vi "数组插入组合.vi"(10 "排序后的一维数组":string[](array[string]), 11 "输入数组":string[][](array[string])) -> (3 "输出结果":string[][](array[string]))   [LabVIEW 2016, in "数据传输系统.lvlib"]
uses:
  <userlib>/_OpenG.lib/array/array.llb/Search 1D Array (String)__ogtk.vi
  <userlib>/_OpenG.lib/array/array.llb/Delete Elements from 2D Array (String)__ogtk.vi
panel:
  out "数组列数":i32
  out "数组":string[][](array[string])
  out "禁用的索引 (列)":i32
  out "Indices of Elements":i32[](array[numeric])
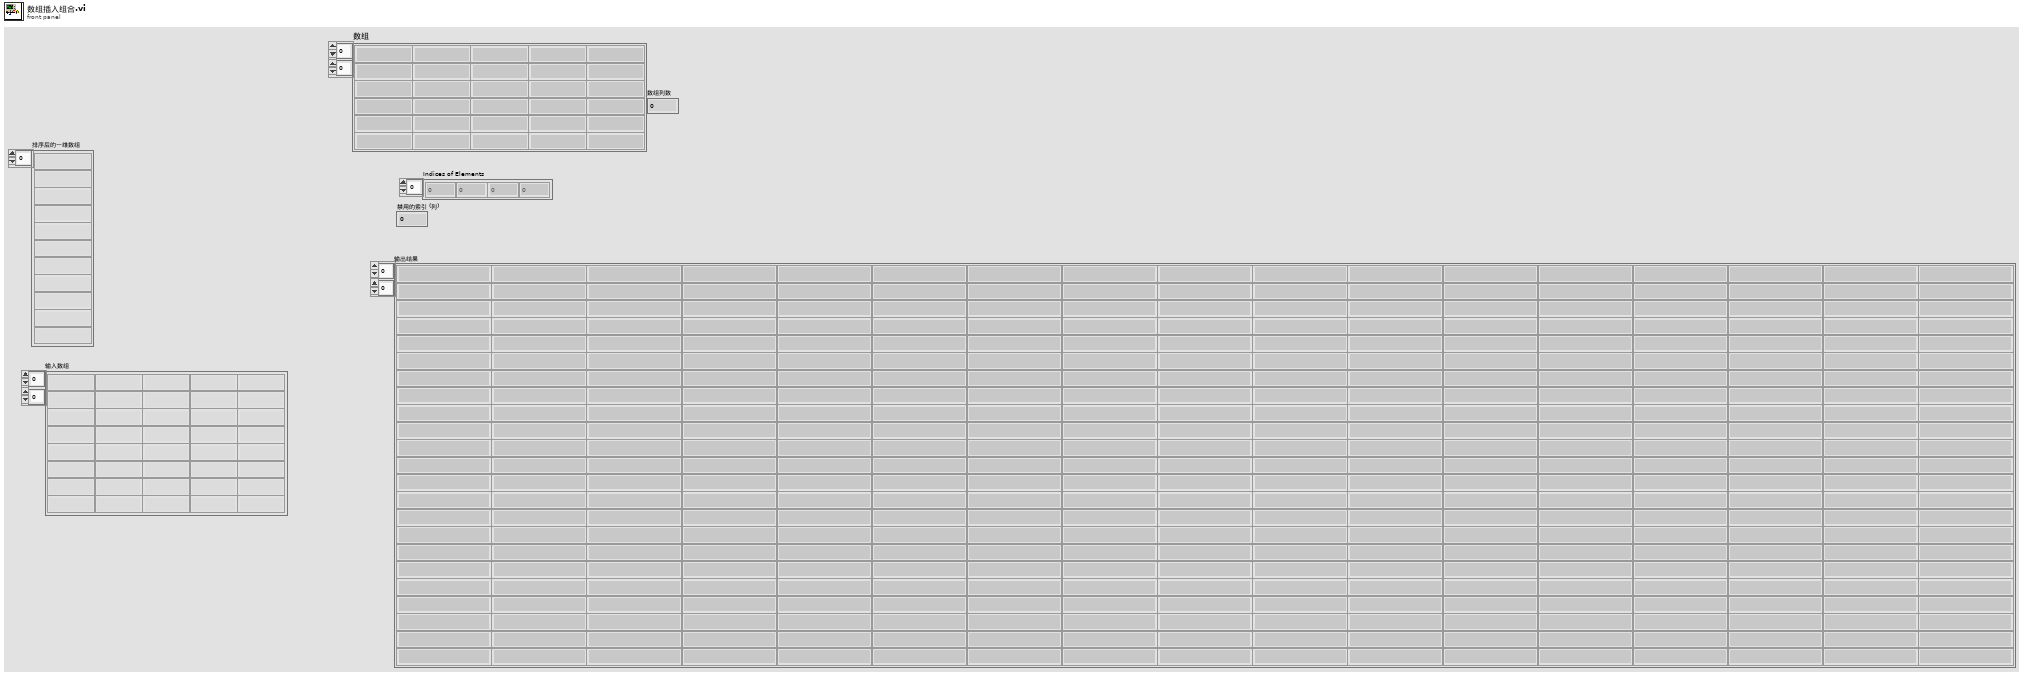
[diagram p1: front panel]
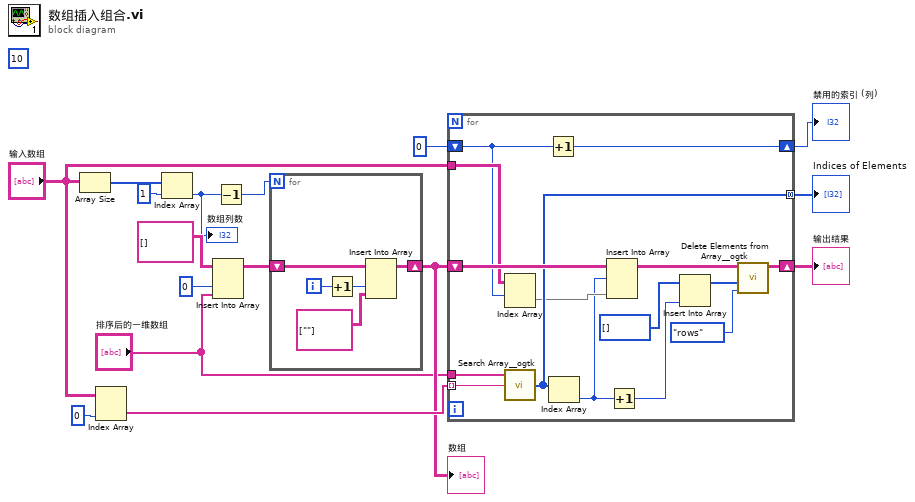
[diagram p0: block diagram]
diagram:
  (unwired) 10
  n1 = Array Size(array="输入数组") -> (size(s)=w5:i32[])
  n2 = Index Array(array="输入数组", index (col)=0 ("禁用的索引 (列)")) -> (element=w13:string[])  [unwired: 1 in]
  n3 = Index Array(array=w5, index=1 ("索引")) -> (element=w2:i32)
  "数组列数" <- w2
  n4 = Insert Into Array(array=string[][] [], index (col)=0 ("禁用的索引 (列)"), new element="排序后的一维数组") -> (w14:string[][])  [unwired: 1 in]
  n5 = Decrement(x=w2) -> (x-1=w3:i32)
  n6 = for {
    N: w3 -> [_]
    shift-right: [w20] -> w9
    shift-left: w14 -> [w21]
    i -> [w19]
    n7 = Increment(x=w19) -> (x+1=w18:i32)
    n8 = Insert Into Array(array=w21, index (col)=w18, new element=string[][] [[""]]) -> (w20:string[][])  [unwired: 1 in]
  }
  "数组" <- w9
  n9 = for {
    tunnel: w13 -> [w36] mode=indexing
    tunnel: "排序后的一维数组" -> [w35]
    tunnel: [w33] -> w12 mode=concatenating
    shift-right: [w27] -> w11
    shift-left: w9 -> [w34]
    shift-right: [w32] -> w10
    shift-left: 0 ("禁用的索引 (列)") -> [w29]
    tunnel: "输入数组" -> [w31]
    n10 = Index Array(array=w31, index (row)=w29) -> (element=w30:string[])  [unwired: 1 in]
    n11 = call-poly <userlib>:"Search Array__ogtk.vi"("Array"=w35, "Element Data"=w36) -> ("Indices of Elements"=w33:i32[])  [unwired: 7 in]
    n12 = Increment(x=w29) -> (x+1=w32:i32)
    n13 = Index Array(array=w33) -> (element=w26:i32)  [unwired: 1 in]
    n14 = Insert Into Array(array=w34, index (row)=w26, new element=w30) -> (w28:string[][])  [unwired: 1 in]
    n15 = Increment(x=w26) -> (x+1=w23:i32)
    n16 = Insert Into Array(array=i32[] [] ("indices"), new element=w23) -> (w24:i32[])  [unwired: 1 in]
    n17 = call-poly <userlib>:"Delete Elements from Array__ogtk.vi"("delete (rows or columns)"=enum16{"rows", "columns"}."rows", "indices"=w24, "array"=w28) -> ("array w/ subset deleted"=w27:string[][])  [unwired: 7 in, 1 out]
  }
  "Indices of Elements" <- w12
  "输出结果" <- w11
  "禁用的索引 (列)" <- w10
